vi "CSDB_Config.get Data.vi"(2 "InstanceName":string, 3 "AttributeName":string, 5 "error in (no error)":errorcluster) -> (16 "Value":string, 19 "error out":errorcluster)   [LabVIEW 2014, in "CSDB_Config.lvlib"]
doc: "Gets the data of an attribute element of an object."
uses:
  CSDB_Config.lvlib
  <vilib>/addons/database/_DB Variant To Data/Database Variant To Data.xnode
  <vilib>/addons/database/NI_Database_API.lvlib
  CSDB_Common/CSDB_Common.lvlib
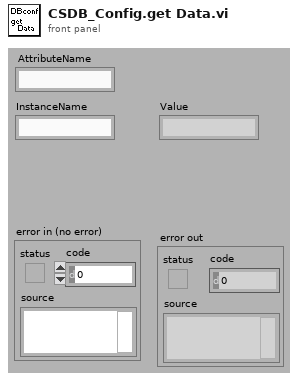
[diagram p1: front panel]
types:
  T1 = typedef "NI_Database_API.lvlib/Conn ObjectReference.ctl" = refnum<k1>
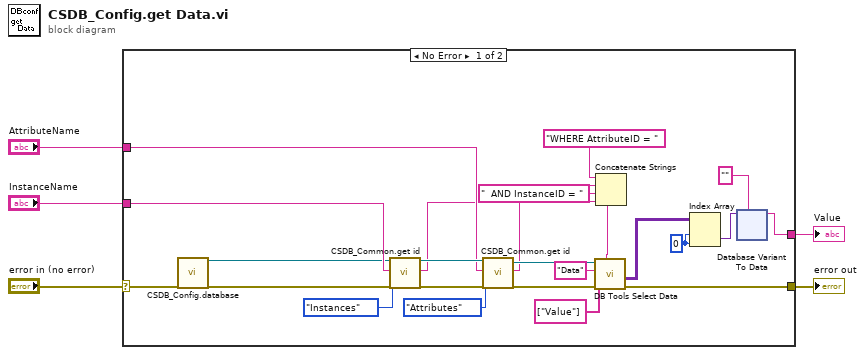
[diagram p0: block diagram]
diagram:
  n1 = case shown="No Error" "error in (no error)" {
    selector: "error in (no error)" -> [w7 w62]
    tunnel: "InstanceName" -> [w26 _]
    tunnel: "AttributeName" -> [w21 _]
    tunnel: [w9 _] -> w3
    tunnel: [w8 w62] -> w2
    frame No Error {
      w29 = 0 ("disabled index (col)")
      n2 = call "CSDB_Config.database.vi"("error in (no error)"=w7) -> ("connectionRef out"=w6:T1, "error out"=w27:errorcluster)  [unwired: 17 in]
      n3 = call "CSDB_Common.get id.vi"("connection reference"=w6, "Class/Attribute/Instance Name"=w26, "Table"=enum16{"Classes", "Attributes", "Instances"}."Instances", "error in (no error)"=w27) -> ("connection reference out"=w24:T1, "ID string"=w16:string, "error out"=w23:errorcluster)  [unwired: 12 in, 1 out]
      n4 = call "CSDB_Common.get id.vi"("connection reference"=w24, "Class/Attribute/Instance Name"=w21, "Table"=enum16{"Classes", "Attributes", "Instances"}."Attributes", "error in (no error)"=w23) -> ("connection reference out"=w20:T1, "ID string"=w17:string, "error out"=w19:errorcluster)  [unwired: 12 in, 1 out]
      n5 = Concatenate Strings("WHERE AttributeID = ", w17, "  AND InstanceID = " ("string"), w16) -> (w15:string)
      n6 = call <vilib>:"DB Tools Select Data.vi"("condition"=w15, "error in (no error)"=w19, "columns"=string[] ["Value"], "table"="Data", "connection reference"=w20) -> ("error out"=w8:errorcluster, "data"=w12:variant[][])  [unwired: 1 in, 1 out]
      n7 = Index Array(array=w12, index (row)=w29, index (col)=w29) -> (element=w11:variant)
      n8 = xnode "Database Variant To Data"("database variant"=w11, "type"="") -> ("data"=w9:string)  [unwired: 1 in, 1 out]
    }
    frame Error {
    }
  }
  "Value" <- w3
  "error out" <- w2
